vi "PPG_ABC.stop ABC.vi"(0 "i ref in":refnum<vi>, 2 "patternGroup":i32, 3 "ms timeout [ms]":i32=10000, 5 "error in (no error)":errorcluster) -> (14 "i ref out":refnum<vi>, 17 "timed out":bool, 19 "error out":errorcluster)   [LabVIEW 2014, in "PPG_ABC.lvlib"]
doc: "Stops execution for the specified pattern group."
uses:
  PPG_ABC.lvlib
  NI_FPGA_PPG/NI_FPGA_PPG.lvlib
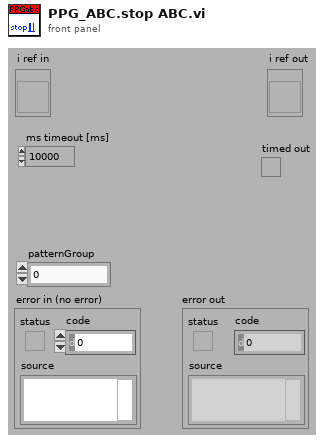
[diagram p1: front panel]
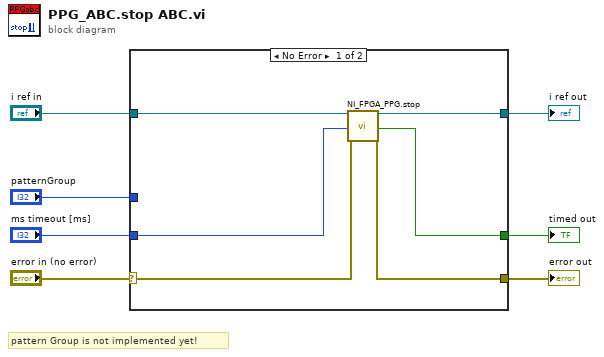
[diagram p0: block diagram]
diagram:
  # "pattern Group is not implemented yet!"
  n1 = case shown="No Error" "error in (no error)" {
    selector: "error in (no error)" -> [w10 w15]
    tunnel: [w9 w15] -> w6
    tunnel: "i ref in" -> [w13 w14]
    tunnel: [w12 w14] -> w4
    tunnel: [w8 _] -> w3
    tunnel: "ms timeout [ms]" -> [w11 _]
    tunnel: "patternGroup" -> [_ _]
    frame No Error {
      n2 = call "NI_FPGA_PPG.stop.vi"("i ref in"=w13, "ms timeout (10000)"=w11, "error in (no error)"=w10) -> ("i ref out"=w12:refnum<vi>, "timed out"=w8:bool, "error out"=w9:errorcluster)  [unwired: 13 in, 1 out]
    }
    frame Error {
    }
  }
  "error out" <- w6
  "i ref out" <- w4
  "timed out" <- w3
